vi "DUT Read.vi"(0 "Digital TSM In":T2, 5 "Number Of Sites":i32, 11 "error in (no error)":errorcluster, 13 "Operation":T1=enum."Read OTP and Timeout") -> (4 "Digital TSM Out":T2, 6 "Per-Site Pass":bool[](array[boolean]), 8 "Per Site Read Data":u8[](array[numeric]), 15 "error out":errorcluster)   [LabVIEW 2020]
uses:
  Instrument Control/Digital/TSM/TSM SSC Digital.ctl
  <vilib>/NI_TestStand_SemiconductorModule/NI_TestStand_Semiconductor_Module.lvlibp/PinMap/Digital Pattern/PinQueryContext/DigitalPatternPinQueryContext.lvclass
  Instrument Control/Digital/SSC Digital/SSC Digital.ctl
  Typedefs/DUT Read Commands.ctl
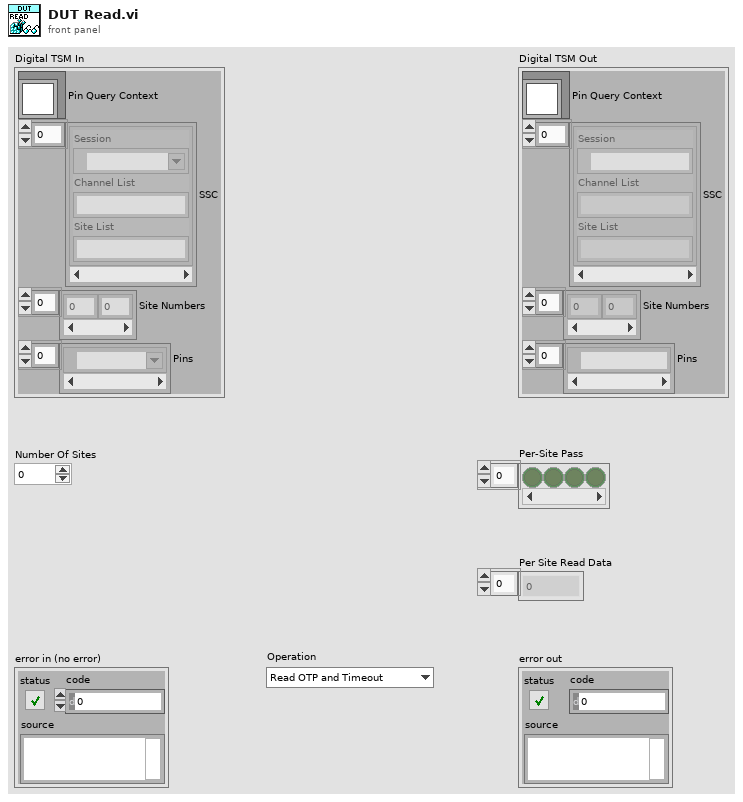
[diagram p1: front panel]
types:
  T1 = typedef "DUT Read Commands.ctl" = enum16{"Read Reg and Timeout", "Read OTP and Timeout"}
  T2 = typedef "TSM SSC Digital.ctl" = cluster{"Pin Query Context":refnum<class "DigitalPatternPinQueryContext.lvclass">, "SSC":T3[], "Site Numbers":i32[], "Pins":tag[]}
  T3 = typedef "SSC Digital.ctl" = cluster{"Session":refnum<k15>, "Channel List":string, "Site List":string}
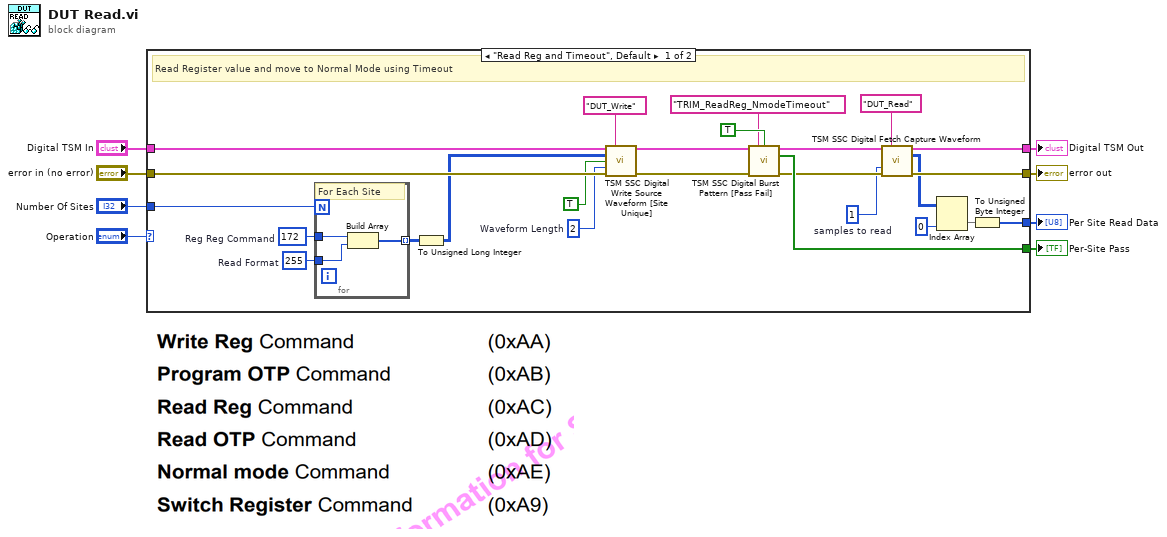
[diagram p0: block diagram]
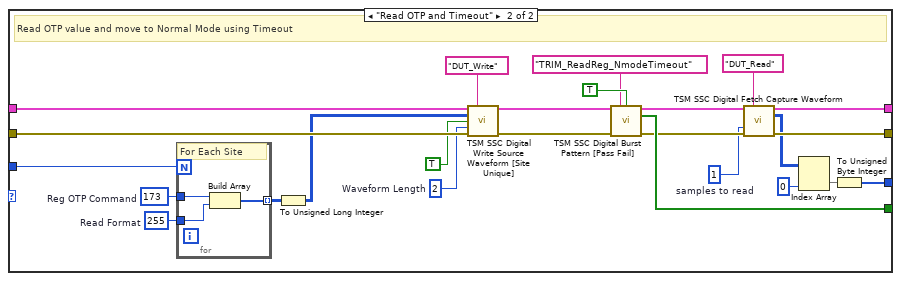
[diagram p2: hidden frame]
diagram:
  n1 = case shown="\"Read Reg and Timeout\", Default" "Operation" {
    tunnel: "Digital TSM In" -> [w32 w60]
    tunnel: "error in (no error)" -> [w31 w59]
    tunnel: "Number Of Sites" -> [w27 w55]
    tunnel: [w23 w51] -> w5
    tunnel: [w20 w48] -> w4
    tunnel: [w19 w47] -> w3
    tunnel: [w14 w42] -> w2
    frame "Read Reg and Timeout", Default {
      w9 = u8 172  # Reg Reg Command
      w18 = 1  # samples to read
      w26 = u8 255  # Read Format
      w29 = 2  # Waveform Length
      # "Read Register value and move to Normal Mode using Timeout"
      n2 = for {
        N: w27 -> [_]
        tunnel: w26 -> [w35]
        tunnel: w9 -> [w36]
        tunnel: [w34] -> w30 mode=indexing
        # "For Each Site"
        n3 = Build Array(w36, w35) -> (w34:u8[])
      }
      n4 = To Unsigned Long Integer(number=w30) -> (unsigned 32bit integer=w13:u32[][])
      n5 = call "TSM SSC Digital Write Source Waveform [Site Unique].vi"("Digital - Sessions in"=w32, "Waveform Name"="DUT_Write", "Per-Site Waveforms"=w13, "Expand to Minimum Size?"=TRUE, "Minimum Size"=w29, "error in"=w31) -> ("Digital - Sessions out"=w24:T2, "error out"=w25:errorcluster)  [unwired: 8 in]
      n6 = call "TSM SSC Digital Burst Pattern [Pass Fail].vi"("Digital TSM In"=w24, "Start Label"="TRIM_ReadReg_NmodeTimeout", "select digital function?"=TRUE, "error in"=w25) -> ("Digital TSM out"=w21:T2, "Per-Site Pass"=w23:bool[], "error out"=w22:errorcluster)  [unwired: 9 in]
      n7 = call "TSM SSC Digital Fetch Capture Waveform.vi"("Digital TSM In"=w21, "Waveform Name"="DUT_Read", "samples to read"=w18, "error in"=w22) -> ("Digital TSM Out"=w20:T2, "Per-Site Waveforms"=w17:u32[][], "error out"=w19:errorcluster)  [unwired: 9 in]
      n8 = Index Array(array=w17, index (col)=0 ("disabled index (col)")) -> (element=w15:u32[])  [unwired: 1 in]
      n9 = To Unsigned Byte Integer(number=w15) -> (unsigned 8bit integer=w14:u8[])
    }
    frame "Read OTP and Timeout" {
      w39 = u8 173  # Reg OTP Command
      w46 = 1  # samples to read
      w54 = u8 255  # Read Format
      w57 = 2  # Waveform Length
      # "Read OTP value and move to Normal Mode using Timeout"
      n10 = for {
        N: w55 -> [_]
        tunnel: w54 -> [w63]
        tunnel: w39 -> [w64]
        tunnel: [w62] -> w58 mode=indexing
        # "For Each Site"
        n11 = Build Array(w64, w63) -> (w62:u8[])
      }
      n12 = To Unsigned Long Integer(number=w58) -> (unsigned 32bit integer=w41:u32[][])
      n13 = call "TSM SSC Digital Write Source Waveform [Site Unique].vi"("Digital - Sessions in"=w60, "Waveform Name"="DUT_Write", "Per-Site Waveforms"=w41, "Expand to Minimum Size?"=TRUE, "Minimum Size"=w57, "error in"=w59) -> ("Digital - Sessions out"=w52:T2, "error out"=w53:errorcluster)  [unwired: 8 in]
      n14 = call "TSM SSC Digital Burst Pattern [Pass Fail].vi"("Digital TSM In"=w52, "Start Label"="TRIM_ReadReg_NmodeTimeout", "select digital function?"=TRUE, "error in"=w53) -> ("Digital TSM out"=w49:T2, "Per-Site Pass"=w51:bool[], "error out"=w50:errorcluster)  [unwired: 9 in]
      n15 = call "TSM SSC Digital Fetch Capture Waveform.vi"("Digital TSM In"=w49, "Waveform Name"="DUT_Read", "samples to read"=w46, "error in"=w50) -> ("Digital TSM Out"=w48:T2, "Per-Site Waveforms"=w45:u32[][], "error out"=w47:errorcluster)  [unwired: 9 in]
      n16 = Index Array(array=w45, index (col)=0 ("disabled index (col)")) -> (element=w43:u32[])  [unwired: 1 in]
      n17 = To Unsigned Byte Integer(number=w43) -> (unsigned 8bit integer=w42:u8[])
    }
  }
  "error out" <- w3
  "Digital TSM Out" <- w4
  "Per-Site Pass" <- w5
  "Per Site Read Data" <- w2
